vi "RSZVB Write Memory Trace Data.vi"(7 "Trace Data":dbl[](array[numeric]) format="%^.3e", 8 "error in (no error)":errorcluster {"code" format="%.0x"}, 9 "No of Points":i32, 10 "Channel (Trace) (1)":i32=1, 11 "VISA session":refnum<visa-resource-name>) -> (0 "error out":errorcluster {"code" format="%.0x"}, 3 "dup VISA session":refnum<visa-resource-name>)   [LabVIEW 2011]
doc: "This VI writes a memory trace data to the instrument.\n\nRemote-control command(s):\nCALCulate<Chn>:DATA SDATa, <data>\nFORMat ASCII\nFORMat REAL,32\nSYSTem:COMMunicate:GPIB:SELF:RTERminator EOI"
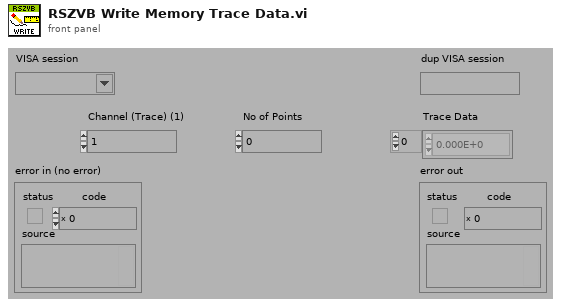
[diagram p1: front panel]
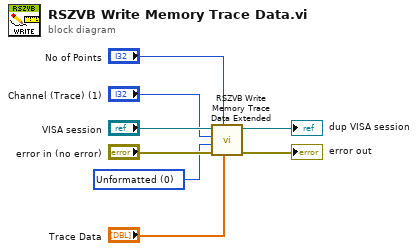
[diagram p0: block diagram]
diagram:
  w1 = 0 items=["Unformatted", "Formatted", "Unformatted With Trace Mathematics"] ("Data Format (0: Unformatted)")
  n1 = call "RSZVB Write Memory Trace Data Extended.vi"("Trace Data"="Trace Data", "No of Points"="No of Points", "error in (no error)"="error in (no error)", "Data Format (0: Unformatted)"=w1, "Channel (Trace) (1)"="Channel (Trace) (1)", "VISA session"="VISA session") -> ("error out"=→"error out":errorcluster, "dup VISA session"=→"dup VISA session":refnum<visa-resource-name>)  [unwired: 4 in]
